vi "Finish.vi"(8 "error in (no error)":errorcluster, 11 "GrabberArms in":refnum<class "GrabberArms.lvclass">) -> (0 "error out":errorcluster, 3 "GrabberArms out":refnum<class "GrabberArms.lvclass">)   [LabVIEW 2013, in "GrabberArms.lvclass"]
uses:
  GrabberArms.lvclass
  System/System.lvclass
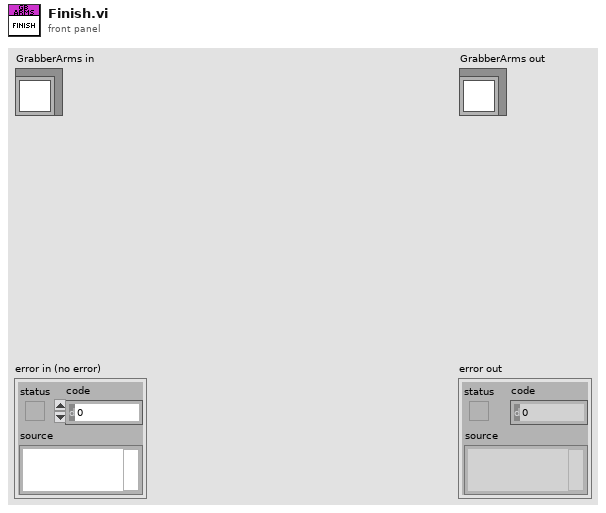
[diagram p1: front panel]
types:
  T1 = typedef "WPI_DigitalInputDevRef.ctl" = cluster{"DevStatus":errorcluster, "DIO Channel":T2, "Digital Module":T3}
  T2 = typedef "FPGA_DIOChannel.ctl" = enum8{"DIO 1", "DIO 2", "DIO 3", "DIO 4", "DIO 5", "DIO 6", "DIO 7", "DIO 8", "DIO 9", "DIO 10", "DIO 11", "DIO 12", "DIO 13", "DIO 14", "Invalid"}
  T3 = typedef "FPGA_TypedefDigitalModule.ctl" = enum16{"Digital Module 1", "Digital Module 2"}
  T4 = typedef "WPI_SolenoidDevRef.ctl" = cluster{"DevStatus":errorcluster, "Solenoid Module":T5, "Forward Solenoid Channel":T6, "Reverse Solenoid Channel":T6}
  T5 = typedef "FPGA_TypedefSolenoidModule.ctl" = enum16{"Solenoid Module 1", "Solenoid Module 2"}
  T6 = typedef "WPI_SolenoidChannel.ctl" = enum8{"Solenoid 1", "Solenoid 2", "Solenoid 3", "Solenoid 4", "Solenoid 5", "Solenoid 6", "Solenoid 7", "Solenoid 8", "Invalid"}
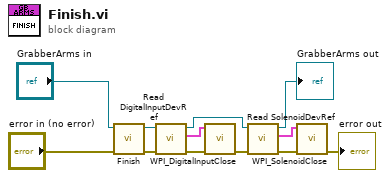
[diagram p0: block diagram]
diagram:
  n1 = call-parent "Finish.vi"("error in (no error)"="error in (no error)", "System in"="GrabberArms in") -> ("error out"=w1:errorcluster, "System out"=w10:refnum<class "GrabberArms.lvclass">)  [unwired: 8 in]
  n2 = call-dynamic "Read DigitalInputDevRef.vi"("error in (no error)"=w1, "GrabberArms in"=w10) -> ("error out"=w2:errorcluster, "DigitalInputDevRef"=w7:T1, "GrabberArms out"=w9:refnum<class "GrabberArms.lvclass">)  [unwired: 7 in]
  n3 = call <vilib>:"WPI_DigitalInputClose.vi"("error in (no error)"=w2, "DigitalInputDevRef"=w7) -> ("error out"=w3:errorcluster)  [unwired: 9 in]
  n4 = call-dynamic "Read SolenoidDevRef.vi"("error in (no error)"=w3, "GrabberArms in"=w9) -> ("error out"=w4:errorcluster, "SolenoidDevRef"=w5:T4, "GrabberArms out"=→"GrabberArms out":refnum<class "GrabberArms.lvclass">)  [unwired: 7 in]
  n5 = call <vilib>:"WPI_SolenoidClose.vi"("error in (no error)"=w4, "SolenoidDevRef"=w5) -> ("error out"=→"error out":errorcluster)  [unwired: 9 in]
